vi "read tag bus value into string.vi"(8 "error in (no error)":errorcluster, 9 "data type":T2, 10 "index":i32, 11 "data table":T1) -> (0 "error out":errorcluster, 3 "Value":string)   [LabVIEW 2013]
uses:
  <vilib>/NI/Tag Bus/tag/Data Type.ctl
  <vilib>/NI/Tag Bus/table/data table.ctl
  <vilib>/NI/Tag Bus/table/data polymorphs/read one/read Double.vi
  <vilib>/NI/Tag Bus/table/data polymorphs/read one/read Single.vi
  <vilib>/NI/Tag Bus/table/data polymorphs/read one/read I64.vi
  <vilib>/NI/Tag Bus/table/data polymorphs/read one/read I32.vi
  <vilib>/NI/Tag Bus/table/data polymorphs/read one/read I16.vi
  <vilib>/NI/Tag Bus/table/data polymorphs/read one/read I8.vi
  <vilib>/NI/Tag Bus/table/data polymorphs/read one/read U64.vi
  <vilib>/NI/Tag Bus/table/data polymorphs/read one/read U32.vi
  <vilib>/NI/Tag Bus/table/data polymorphs/read one/read U16.vi
  <vilib>/NI/Tag Bus/table/data polymorphs/read one/read U8.vi
  <vilib>/NI/Tag Bus/table/data polymorphs/read one/read String.vi
  <vilib>/NI/Tag Bus/table/data polymorphs/read one/read Boolean.vi
  <vilib>/NI/Tag Bus/table/data table.lvlib
  <vilib>/NI/Tag Bus/tag/tag descriptor.lvclass
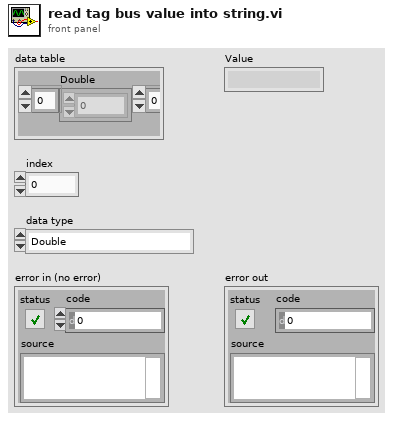
[diagram p1: front panel]
types:
  T1 = typedef "tag bus.lvlib/data table.lvlib/data table.ctl" = cluster{"Double":dbl[], "Single":sgl[], "I64":i64[], "I32":i32[], "I16":i16[], "I8":i8[], "U64":u64[], "U32":u32[], "U16":u16[], "U8":u8[], "Boolean":bool[], "String":string[], "Array of Double":cluster{"DBL Array":dbl[]}[], "Array of Single":cluster{"SGL Array":sgl[]}[], "Array of I64":cluster{"I64 Array":i64[]}[], "Array of I32":cluster{"I32 Array":i32[]}[], "Array of I16":cluster{"I16 Array":i16[]}[], "Array of I8":cluster{"I8 Array":i8[]}[], "Array of U64":cluster{"U64 Array":u64[]}[], "Array of U32":cluster{"U32 Array":u32[]}[], "Array of U16":cluster{"U16 Array":u16[]}[], "Array of U8":cluster{"U8 Array":u8[]}[], "Array of Boolean":cluster{"Boolean Array":bool[]}[], "Array of String":cluster{"String Array":string[]}[]}
  T2 = typedef "tag bus.lvlib/tag descriptor.lvclass/Data Type.ctl" = enum16{"Double", "Single", "I64", "I32", "I16", "I8", "U64", "U32", "U16", "U8", "Boolean", "String", "Array of Double", "Array of Single", "Array of I64", "Array of I32", "Array of I16", "Array of I8", "Array of U64", "Array of U32", "Array of U16", "Array of U8", "Array of Boolean", "Array of String"}
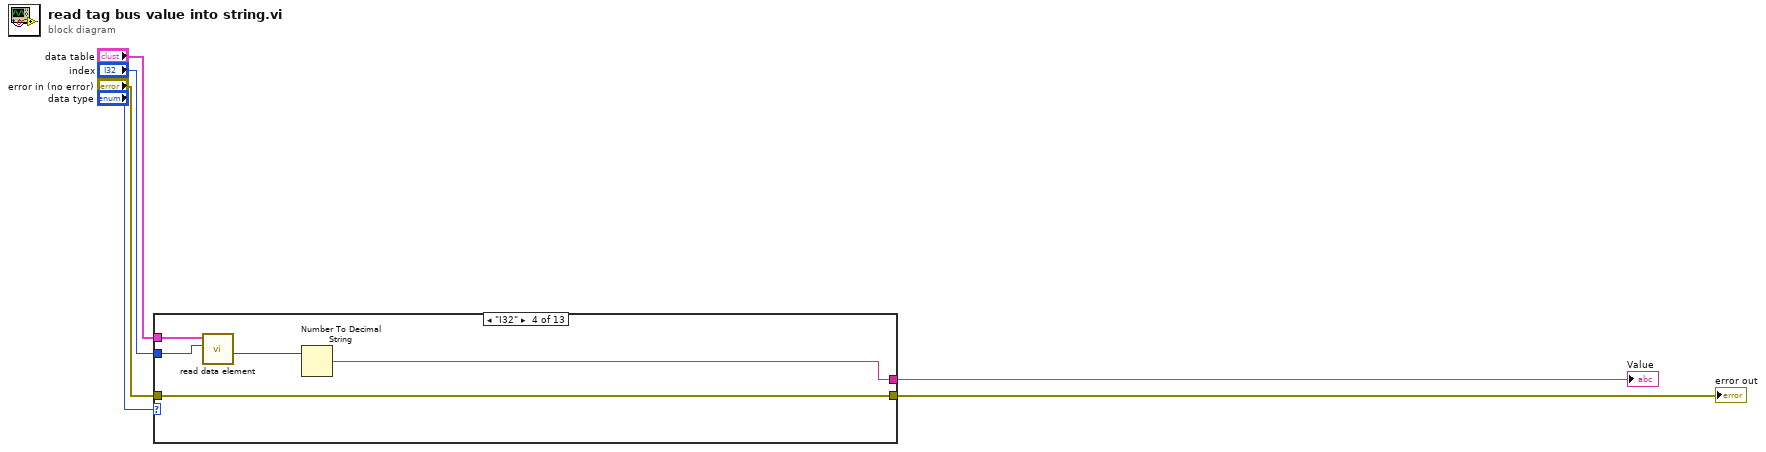
[diagram p0: block diagram]
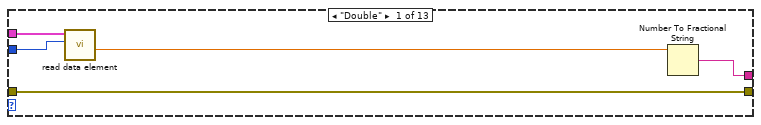
[diagram p2: hidden frame]
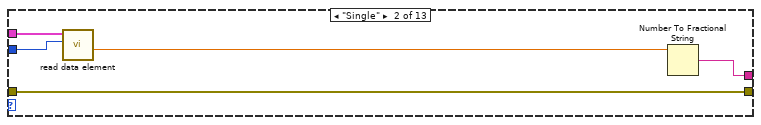
[diagram p3: hidden frame]
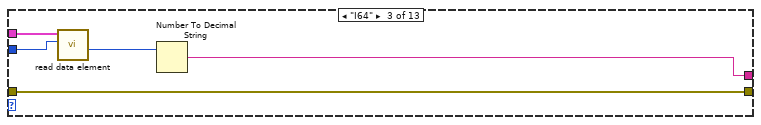
[diagram p4: hidden frame]
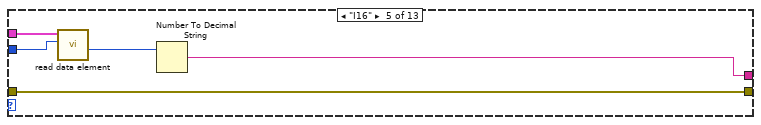
[diagram p5: hidden frame]
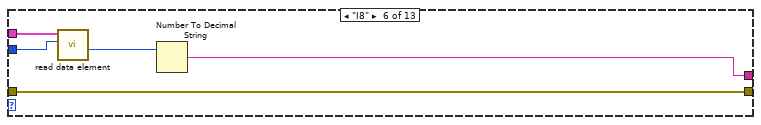
[diagram p6: hidden frame]
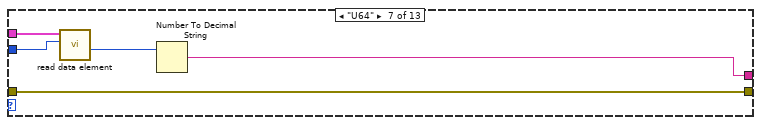
[diagram p7: hidden frame]
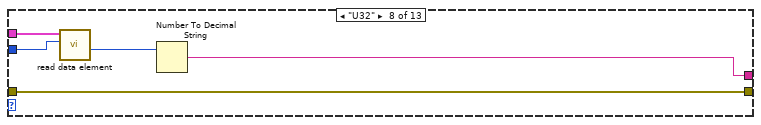
[diagram p8: hidden frame]
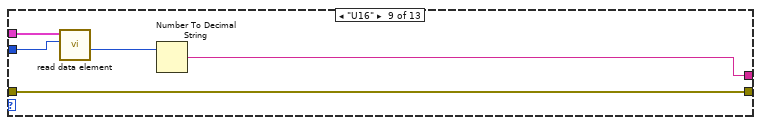
[diagram p9: hidden frame]
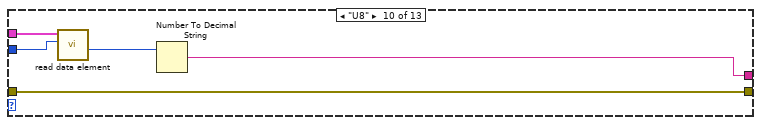
[diagram p10: hidden frame]
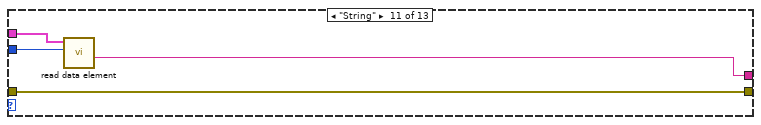
[diagram p11: hidden frame]
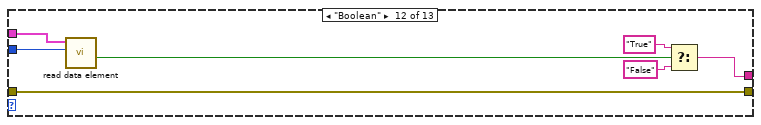
[diagram p12: hidden frame]
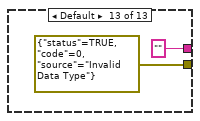
[diagram p13: hidden frame]
diagram:
  n1 = case shown="\"I32\"" "data type" {
    tunnel: [w11 w14 w20 w25 w30 w35 w40 w45 w50 w55 w57 w64 "" ("Value")] -> w1
    tunnel: [w10 w13 w21 w26 w31 w36 w41 w46 w51 w56 w60 w67 errorcluster {"status"=TRUE, "code"=0, "source"="Invalid Data Type"} ("error out")] -> w3
    tunnel: "error in (no error)" -> [w10 w13 w21 w26 w31 w36 w41 w46 w51 w56 w60 w67 _]
    tunnel: "data table" -> [w9 w16 w19 w24 w29 w34 w39 w44 w49 w54 w59 w62 _]
    tunnel: "index" -> [w8 w12 w18 w23 w28 w33 w38 w43 w48 w53 w58 w63 _]
    frame "Double" {
      n2 = call-poly <vilib>:"read data element.vi"("index"=w8, "data table in"=w9) -> ("value"=w7:dbl)  [unwired: 8 in, 1 out]
      n3 = Number To Fractional String(number=w7) -> (F-format string=w11:string)  [unwired: 3 in]
    }
    frame "Single" {
      n4 = call-poly <vilib>:"read data element.vi"("index"=w12, "data table in"=w16) -> ("value"=w15:sgl)  [unwired: 8 in, 1 out]
      n5 = Number To Fractional String(number=w15) -> (F-format string=w14:string)  [unwired: 3 in]
    }
    frame "I64" {
      n6 = call-poly <vilib>:"read data element.vi"("index"=w18, "data table in"=w19) -> ("value"=w17:i64)  [unwired: 8 in, 1 out]
      n7 = Number To Decimal String(number=w17) -> (decimal integer string=w20:string)  [unwired: 1 in]
    }
    frame "I32" {
      n8 = call-poly <vilib>:"read data element.vi"("index"=w23, "data table in"=w24) -> ("value"=w22:i32)  [unwired: 8 in, 1 out]
      n9 = Number To Decimal String(number=w22) -> (decimal integer string=w25:string)  [unwired: 1 in]
    }
    frame "I16" {
      n10 = call-poly <vilib>:"read data element.vi"("index"=w28, "data table in"=w29) -> ("value"=w27:i16)  [unwired: 8 in, 1 out]
      n11 = Number To Decimal String(number=w27) -> (decimal integer string=w30:string)  [unwired: 1 in]
    }
    frame "I8" {
      n12 = call-poly <vilib>:"read data element.vi"("index"=w33, "data table in"=w34) -> ("value"=w32:i8)  [unwired: 8 in, 1 out]
      n13 = Number To Decimal String(number=w32) -> (decimal integer string=w35:string)  [unwired: 1 in]
    }
    frame "U64" {
      n14 = call-poly <vilib>:"read data element.vi"("index"=w38, "data table in"=w39) -> ("value"=w37:u64)  [unwired: 8 in, 1 out]
      n15 = Number To Decimal String(number=w37) -> (decimal integer string=w40:string)  [unwired: 1 in]
    }
    frame "U32" {
      n16 = call-poly <vilib>:"read data element.vi"("index"=w43, "data table in"=w44) -> ("value"=w42:u32)  [unwired: 8 in, 1 out]
      n17 = Number To Decimal String(number=w42) -> (decimal integer string=w45:string)  [unwired: 1 in]
    }
    frame "U16" {
      n18 = call-poly <vilib>:"read data element.vi"("index"=w48, "data table in"=w49) -> ("value"=w47:u16)  [unwired: 8 in, 1 out]
      n19 = Number To Decimal String(number=w47) -> (decimal integer string=w50:string)  [unwired: 1 in]
    }
    frame "U8" {
      n20 = call-poly <vilib>:"read data element.vi"("index"=w53, "data table in"=w54) -> ("value"=w52:u8)  [unwired: 8 in, 1 out]
      n21 = Number To Decimal String(number=w52) -> (decimal integer string=w55:string)  [unwired: 1 in]
    }
    frame "String" {
      n22 = call-poly <vilib>:"read data element.vi"("index"=w58, "data table in"=w59) -> ("value"=w57:string)  [unwired: 8 in, 1 out]
    }
    frame "Boolean" {
      n23 = call-poly <vilib>:"read data element.vi"("index"=w63, "data table in"=w62) -> ("value"=w61:bool)  [unwired: 8 in, 1 out]
      n24 = Select(t="True", s=w61, f="False") -> (s? t:f=w64:string)
    }
    frame Default {
    }
  }
  "error out" <- w3
  "Value" <- w1
